vi "PIV_Pixel.vi"(8 "error in (no error)":errorcluster, 11 "PIV params":T2={"t"=path "/Users/crogers/Desktop/PIV/ezgif-split/frame_0_delay-0.14s.jpg", "t + dt"=path "/Users/crogers/Desktop/PIV/ezgif-split/frame_1_delay-0.14s.jpg", "PIV params"={"window size"=32, "search size"=38, "overlap"=17}}) -> (0 "error out":errorcluster={"status"=TRUE, "code"=1671, "source"="Python Node in PIV_Pixel.vi->LabVIEW_GUI.vi<APPEND>\n\nModule Path: /Users/crogers/Desktop/PIV/LabVIEW/subs/code.py\nFunction Name: piv\nPython returned the following error: <class 'OSError'>\nImageIO does not generally support reading folders. Limited support may be available via specific plugins. Specify the plugin explicitly using the `plugin` kwarg, e.g. `plugin='DICOM'`\n\n\n Call Stack information:\n['Traceback (most recent call last):\n', '  File \"/Users/crogers/Desktop/PIV/LabVIEW/subs/code.py\", line 8, in piv\n    frame_a = tools.imread(path_t)\n', '  File \"/Users/crogers/Library/Python/3.10/lib/python/site-packages/openpiv/tools.py\", line 337, in imread\n    im = _imread(filename)\n', '  File \"/Users/crogers/Library/Python/3.10/lib/python/site-packages/imageio/v3.py\", line 53, in imread\n    with imopen(uri, \"r\", **plugin_kwargs) as img_file:\n', '  File \"/Users/crogers/Library/Python/3.10/lib/python/site-packages/imageio/core/imopen.py\", line 223, in imopen\n    raise err_type(err_msg)\n', \"OSError: ImageIO does not generally support reading folders. Limited support may be available via specific plugins. Specify the plugin explicitly using the `plugin` kwarg, e.g. `plugin='DICOM'`\n\"]"}, 3 "pixels":T1={"x"=[[249.30535937373418, 248.42902364889454, 249.76279948299583, 247.41594341275038, 249.1115257279782, 247.78798944960093, 250.12043012406355, 247.87808352883224, 248.34885972253088, 249.7914207911112, 247.77762730848636, 249.1512614353793, 249.75511132386535, 250.2039453992136, 251.0671966033442, 249.57524164043096], [250.3340434377881, 250.00147110119926, 248.9863350898821, 248.5777445935735, 248.8999381795624, 248.0999411317878, 250.1052613689504, 248.91784014699442, 248.86156436587453, 250.04009873380096, 249.0256554262938, 248.65809383974363, 249.6866801516841, 250.34192499126266, 248.82795554993143, 249.0061437567773], [249.8379771192706, 249.42545268743535, 249.99132868734347, 248.92736756105637, 248.81643484942745, 249.3310863564142, 250.15105027103033, 249.12989134088602, 249.04454959724643, 247.59519201729674, 249.25833529503674, 247.47331898457645, 248.1888431064803, 250.79040549336878, 249.4526081113374, 249.6336800524876], [248.6980668234578, 248.54570865688697, 246.7725657136647, 249.35812326520707, 248.89034255886847, 246.4523690408173, 250.0452232403072, 249.550444871314, 249.9765476901514, 248.7568049322972, 248.6401612231491, 249.79883085797923, 249.40130797289405, 246.5629890714208, 247.80685370459122, 248.80462667572783], [250.01488921592187, 250.09153234704317, 248.9121711813194, 249.0997960432928, 248.23464430329008, 248.5390445092607, 250.14199554538584, 249.79526944527598, 249.15547166133257, 248.42913742312317, 248.66649765678002, 249.98783358463044, 249.3122662178276, 247.46275715637935, 247.09281127164536, 249.14196469060883], [248.4814726325146, 250.32578418378327, 252.73547131633674, 249.2578741433366, 248.12604140003066, 249.92341822045444, 250.0776499368854, 248.399064003398, 246.77201099675497, 248.27129179389703, 250.55497705596306, 249.65928326586936, 249.59825543346153, 247.44042616526, 248.20411140311407, 248.28014466979678], [248.00737255317583, 250.54707211705906, 249.21162645077857, 248.25886125408834, 248.0387539726566, 248.9153012638658, 250.18519850567776, 247.22467702968024, 249.76466629672095, 249.2556306748364, 250.02396374442702, 249.65051950062963, 250.4965660861888, 248.0925292927269, 248.91946592643953, 248.2637943515181], [246.1821494594906, 249.33082934098553, 248.94094393264493, 249.04158620653422, 249.26011732344762, 249.6661630920858, 248.34537482290315, 249.32958002145983, 248.44306056595542, 249.60284556401166, 249.11509294896507, 249.91933165248471, 248.13237489941073, 250.05627478689743, 248.8303136103349, 249.21198396258842], [247.40937679664955, 249.75749896985545, 248.32387807731334, 248.95535998273797, 250.07904312089906, 248.94164695256754, 247.77049810385864, 247.87385923341975, 248.15868824776928, 249.5424691779508, 248.67114136119247, 248.60481452263753, 247.09329148360536, 250.04657782089552, 247.76622030389302, 249.74825372082137], [248.40649315075004, 249.50680197039077, 249.01580784201263, 248.08513546511418, 250.23552350579513, 248.0561485178251, 249.0645116452157, 248.95113258123106, 251.75665115657733, 249.3997539918615, 248.66201521458854, 248.85160979570387, 248.38535817779288, 248.46760230981192, 247.46861084204957, 249.0122244330493], [249.14754561374613, 251.02569476688643, 249.8361169122564, 247.93392565584398, 249.95930525996766, 248.6162386371012, 249.08361536717862, 249.87630209464092, 249.48931646095573, 249.14607663576936, 248.62804527022283, 249.4249745322186, 248.7380918318621, 249.3604159325276, 248.72143788477564, 249.21304894216297], [248.35312686069207, 249.58820056157424, 248.3560103286516, 249.56629318575628, 249.59362672842414, 249.60331244219543, 249.10441364055487, 248.7328086777035, 248.89866953363116, 247.97866927062663, 249.3307073073744, 250.2239182398913, 249.16142037868028, 249.0563871396553, 249.4949006882887, 249.51436619145983]], "y"=[[0.8977283953687021, 0.6341863158832339, 0.9906547908510532, 3.106737289418504, 1.1821140984592304, 0.3751409283520246, 1.3818005864610683, -0.600121285455657, 0.6357268023560181, 0.845736566623323, -0.3731915769522587, -2.199033492516911, -0.21423581669690606, -0.3347594797784126, 1.1698087519270928, 1.566926374462696], [0.8965659508572088, 1.9437460996389433, 0.6224521757415502, -0.7217534453584307, 1.2037735939395944, 3.040914323466559, -0.3832771542393587, 0.15343686298088244, 0.997187747340611, 1.0527446150261355, 1.509697354230255, -2.1701091702073683, -2.2892314742890107, -0.6124409762401584, 1.25779577345142, 2.435950520643182], [-0.020908984575918055, 0.808132754103319, 1.5727649641668506, -0.45296926287363704, -1.208464478259863, -0.506959993186129, -0.5947669843271441, -0.975848708630167, -0.6421905816051066, -0.3987990096717908, -1.4070992684436234, -2.261505865838487, 0.06639054799464361, -1.1695814137185678, -0.3675269379222357, -0.2648923594257724], [0.3109771407276085, 0.5159494570786904, -1.4163299456319223, 0.07102651210981747, -1.2851252719297435, 0.10599760454645946, 0.7367107969054487, -0.16784210153293344, 0.27284316723275026, 0.4596314702594029, -0.4132105382968376, 2.593889260250748, 0.45294607371371143, -1.933834795200795, -1.0096684879789208, -0.15903235101450974], [0.23855007598676536, -1.9955308986860487, -1.3984666925978217, 0.48058552946130817, -0.015174367898751484, -0.7671366273104496, -0.8535820787912485, -0.7955505153384834, -1.017646873453515, -0.16739074452090108, 0.3648306981711258, 0.9307679362089871, 1.562958664327141, -0.04485662689486247, -0.23357418783209738, -0.6035663171106265], [0.013829448925584131, -1.9358349688371135, -1.4695962162198484, 0.5947964198860234, 0.2776392219589141, -0.22785775633131777, -0.15131917925703675, -0.4153649199674092, 0.4466333336464956, 0.25066493260030853, 0.35528947786236387, 1.3103000240386464, -0.2140304542018967, 0.12133392372160046, -0.49735044708949516, -0.2563433389042302], [2.0066903381980694, 2.794937422495103, 1.3981438682431957, 1.32543349324159, 0.022886535372457217, -0.9432851645218676, 0.0465564365104143, -0.9851058035259541, 0.8804035526296161, 1.2072293754869179, 0.42874909844545783, 1.7652653432293164, 0.47987536243230267, 0.26211844447008303, 0.6477767135804058, 1.191164256120203], [2.1410994418467055, 1.1177174463222528, 1.6983097882253162, 0.7617018915272666, 1.8895481438185868, -2.3308329687965923, 0.44458370084541343, 3.4411635098964055, 0.4202762082936573, -0.7767577642360024, -0.35753351457277205, -0.3741674249379656, 0.22728149074637827, -0.08923809505407831, 0.6029678418080664, 1.8102033968000697], [0.40552532193807167, 0.38050416917148056, 2.9728620478863377, 0.5848556588837539, 0.034000271349654554, -1.0697151619861955, -0.789201625615199, 0.3424590331110977, -0.014991496301952623, 0.1816448684692773, 0.16450838718995442, -0.8527519183298082, 0.5973103946411484, -0.21929086910912332, -0.2522634668837398, -0.5496729535634515], [-1.0784341723001134, 0.6385179489532433, 0.2624355393884059, 0.7800818345774729, -0.20223131443852793, -0.8799262477261038, 1.0814261425313276, 0.01896169162503014, -1.4323416215907159, -1.1447899618840296, 1.2953715679074662, 1.8011306347966993, -3.59547558301756, -1.51425732727688, -0.3005536713368784, -0.8495876802721014], [-0.48529100956749005, 3.7535484211289827, 0.4716731565341803, -0.16691798810644087, -1.3274681438865343, 1.4127784125875564, 2.503009927378308, 0.6744977470081182, 0.6289537982436144, 0.5592686551672443, -0.4793140551587527, 0.8966787006954746, 2.8181705852389882, 0.8982376832276984, 0.8024882650817133, 0.36402627005394095], [0.3348076271773692, 0.5833426717044787, 0.6325826470115814, -1.2167231134881717, 0.2408720624673677, -0.5408144273093995, 0.061549655902659595, 0.1198560631205936, 0.4155138438417083, -0.07385728581841278, 1.0016705373303125, -0.8491469124310314, -1.0571250384478148, 0.27765360370057834, 1.3863896930917718, 1.2780985374410747]], "u"=[[3.654057076523203, 3.906689254019018, 4.3499249727354785, 2.9769797253005232, 4.1985261262312195, 4.53911201630744, 3.6142265703335354, 4.545410360329742, 4.275176542616173, 3.9800504580894107, 3.945780644550432, 4.142828981573519, 3.997707165543276, 2.9923959435801497, 3.4106969202636495, 4.999245369266826], [4.721876610704807, 2.7791735544418565, 4.04797726724709, 3.1329268783475097, 4.706557050441488, 4.762468241690385, 3.039882623852986, 5.037812189846022, 3.357303836725008, 3.4488968279603935, 3.924508990313546, 4.201571037936669, 4.017913649448239, 4.3435322093850495, 4.387257019168252, 3.9180399717234993], [4.511693109203351, 3.6612724986035223, 4.269814446623989, 4.218697651581058, 4.807320057264706, 4.009377669328912, 4.405847778900064, 4.123688871016016, 3.784958247444461, 3.721978603867669, 4.353352122442394, 3.440608423789492, 4.8110182227292855, 3.909255097098531, 2.9020670167480147, 3.9050361810819143], [3.40465714069752, 3.9326981284321607, 4.0120727049173555, 3.7856505254893382, 3.7262750849724515, 2.9831152945719106, 3.7097179258624338, 4.35106035811602, 3.688332772188065, 3.747091966193779, 4.11025427675998, 3.9656181661692327, 2.9327313456835538, 4.150277635628887, 3.3765339532142065, 4.153106429159354], [3.387574609047479, 2.7699051515052755, 4.107458409125639, 4.471004094839486, 3.630386589969853, 3.7522818291832034, 4.592562274282968, 4.942019544439905, 3.6758264536017187, 5.090556637656444, 4.392992010857408, 3.7361463084414557, 2.644273868496813, 4.235012879773729, 4.017292315069722, 4.615785073786853], [4.845808184377554, 4.439541657576462, 2.897607886694547, 3.4661358674422065, 4.114576567616225, 4.2981580154498165, 4.45289017699371, 3.1067911933459214, 3.9731156019297735, 4.967565161826359, 4.274648262718975, 3.340537457109602, 4.007790619783492, 3.0484698597456186, 3.0902877440316217, 3.46977172973948], [4.105784905034725, 4.367232594403088, 3.4482894359240186, 3.519447403701663, 4.1592118776098825, 4.452636112938493, 4.402274236537246, 3.8791091835025098, 4.280101204874112, 4.097948666253696, 3.7883707470561188, 4.824890734154082, 4.952756144044697, 4.431182097404486, 4.243449943530994, 4.838679874357956], [3.400017358160556, 4.131421512821141, 4.1341151479233815, 3.868056363739919, 4.114722937313372, 3.182209432540521, 4.614370434260993, 4.411780339295759, 3.7355216305789054, 4.594274939159283, 4.491351839228378, 4.3193175610411325, 3.9283857185683773, 4.793911290126535, 4.649497598758955, 4.3396642398318335], [3.516007589124258, 4.196871268766618, 3.1728676439509176, 3.420084255337708, 4.592612630487026, 3.4822313601511596, 4.212353707965761, 5.4044957155037405, 4.095326795337716, 4.74614522754851, 5.01002718991552, 4.34430597630962, 4.3788685927631015, 4.9484451474366296, 3.6714296162586293, 3.410028692944248], [4.114243758496789, 3.342175456154506, 4.0764258974027605, 3.7136810067221804, 4.477618301281832, 4.208710770028269, 4.001606540014744, 3.657763910976016, 3.8103669626271897, 4.458090941819041, 3.891518974609637, 4.030571187954858, 2.728773248181442, 4.326154268416609, 4.733378911855885, 4.609860862498076], [3.7273513628033554, 2.4461192162266197, 3.9403444180392935, 4.236797064872377, 3.5225832678408047, 3.9117408717259883, 3.788069871625027, 4.554181400594344, 3.475295946618708, 3.288247776778453, 4.779964981541216, 3.6684037998946164, 3.1969710305814667, 3.7169385489979185, 3.872757705734433, 3.64012465662325], [3.4516528893089995, 4.387557930694406, 3.994367234165161, 4.086502040222127, 3.302726609880943, 4.115138490819219, 4.143240057429105, 4.669707669133866, 3.7284189048703174, 4.039756580842941, 2.557244072683501, 3.6402231851260347, 4.066441820254696, 4.519502569432314, 4.11575653582123, 4.385562395092346]], "v"=[[21.0, 42.0, 63.0, 84.0, 105.0, 126.0, 147.0, 168.0, 189.0, 210.0, 231.0, 252.0, 273.0, 294.0, 315.0, 336.0], [21.0, 42.0, 63.0, 84.0, 105.0, 126.0, 147.0, 168.0, 189.0, 210.0, 231.0, 252.0, 273.0, 294.0, 315.0, 336.0], [21.0, 42.0, 63.0, 84.0, 105.0, 126.0, 147.0, 168.0, 189.0, 210.0, 231.0, 252.0, 273.0, 294.0, 315.0, 336.0], [21.0, 42.0, 63.0, 84.0, 105.0, 126.0, 147.0, 168.0, 189.0, 210.0, 231.0, 252.0, 273.0, 294.0, 315.0, 336.0], [21.0, 42.0, 63.0, 84.0, 105.0, 126.0, 147.0, 168.0, 189.0, 210.0, 231.0, 252.0, 273.0, 294.0, 315.0, 336.0], [21.0, 42.0, 63.0, 84.0, 105.0, 126.0, 147.0, 168.0, 189.0, 210.0, 231.0, 252.0, 273.0, 294.0, 315.0, 336.0], [21.0, 42.0, 63.0, 84.0, 105.0, 126.0, 147.0, 168.0, 189.0, 210.0, 231.0, 252.0, 273.0, 294.0, 315.0, 336.0], [21.0, 42.0, 63.0, 84.0, 105.0, 126.0, 147.0, 168.0, 189.0, 210.0, 231.0, 252.0, 273.0, 294.0, 315.0, 336.0], [21.0, 42.0, 63.0, 84.0, 105.0, 126.0, 147.0, 168.0, 189.0, 210.0, 231.0, 252.0, 273.0, 294.0, 315.0, 336.0], [21.0, 42.0, 63.0, 84.0, 105.0, 126.0, 147.0, 168.0, 189.0, 210.0, 231.0, 252.0, 273.0, 294.0, 315.0, 336.0], [21.0, 42.0, 63.0, 84.0, 105.0, 126.0, 147.0, 168.0, 189.0, 210.0, 231.0, 252.0, 273.0, 294.0, 315.0, 336.0], [21.0, 42.0, 63.0, 84.0, 105.0, 126.0, 147.0, 168.0, 189.0, 210.0, 231.0, 252.0, 273.0, 294.0, 315.0, 336.0]], "Sig2noise"=[[24.0, 24.0, 24.0, 24.0, 24.0, 24.0, 24.0, 24.0, 24.0, 24.0, 24.0, 24.0, 24.0, 24.0, 24.0, 24.0], [45.0, 45.0, 45.0, 45.0, 45.0, 45.0, 45.0, 45.0, 45.0, 45.0, 45.0, 45.0, 45.0, 45.0, 45.0, 45.0], [66.0, 66.0, 66.0, 66.0, 66.0, 66.0, 66.0, 66.0, 66.0, 66.0, 66.0, 66.0, 66.0, 66.0, 66.0, 66.0], [87.0, 87.0, 87.0, 87.0, 87.0, 87.0, 87.0, 87.0, 87.0, 87.0, 87.0, 87.0, 87.0, 87.0, 87.0, 87.0], [108.0, 108.0, 108.0, 108.0, 108.0, 108.0, 108.0, 108.0, 108.0, 108.0, 108.0, 108.0, 108.0, 108.0, 108.0, 108.0], [129.0, 129.0, 129.0, 129.0, 129.0, 129.0, 129.0, 129.0, 129.0, 129.0, 129.0, 129.0, 129.0, 129.0, 129.0, 129.0], [150.0, 150.0, 150.0, 150.0, 150.0, 150.0, 150.0, 150.0, 150.0, 150.0, 150.0, 150.0, 150.0, 150.0, 150.0, 150.0], [171.0, 171.0, 171.0, 171.0, 171.0, 171.0, 171.0, 171.0, 171.0, 171.0, 171.0, 171.0, 171.0, 171.0, 171.0, 171.0], [192.0, 192.0, 192.0, 192.0, 192.0, 192.0, 192.0, 192.0, 192.0, 192.0, 192.0, 192.0, 192.0, 192.0, 192.0, 192.0], [213.0, 213.0, 213.0, 213.0, 213.0, 213.0, 213.0, 213.0, 213.0, 213.0, 213.0, 213.0, 213.0, 213.0, 213.0, 213.0], [234.0, 234.0, 234.0, 234.0, 234.0, 234.0, 234.0, 234.0, 234.0, 234.0, 234.0, 234.0, 234.0, 234.0, 234.0, 234.0], [255.0, 255.0, 255.0, 255.0, 255.0, 255.0, 255.0, 255.0, 255.0, 255.0, 255.0, 255.0, 255.0, 255.0, 255.0, 255.0]]})   [LabVIEW 2025]
uses:
  PIV_params.ctl
  PIV_velocities.ctl
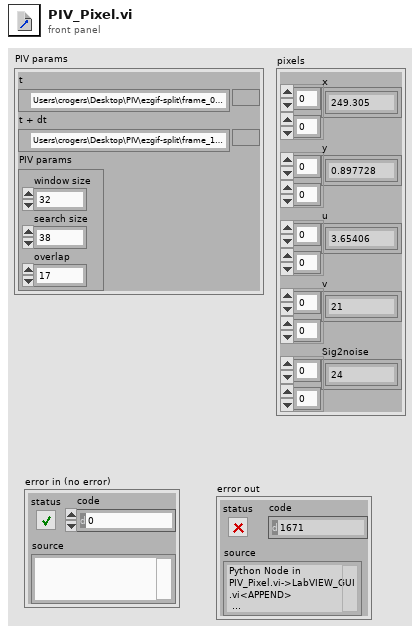
[diagram p1: front panel]
types:
  T1 = typedef "PIV_velocities.ctl" = cluster{"x":dbl[][], "y":dbl[][], "u":dbl[][], "v":dbl[][], "Sig2noise":dbl[][]}
  T2 = typedef "PIV_params.ctl" = cluster{"t":path, "t + dt":path, "PIV params":cluster{"window size":i16, "search size":i16, "overlap":i16}}
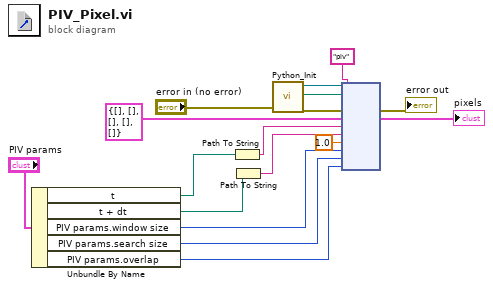
[diagram p0: block diagram]
diagram:
  n1 = Unbundle By Name("PIV params") -> ("t"=w5:path, "t + dt"=w4:path, "PIV params.window size"=w9:i16, "PIV params.search size"=w8:i16, "PIV params.overlap"=w7:i16)
  n2 = Path To String(path=w5) -> (string=w11:string)
  n3 = Path To String(path=w4) -> (string=w10:string)
  n4 = call "Python_Init.vi"("error in (no error)"="error in (no error)") -> ("Refnum out"=w16:refnum<k35>, "code"=w13:path, "error out"=w17:errorcluster)  [unwired: 3 in]
  n5 = node(w16, w13, "piv" ("function name"), w17, T1 {"x"=[], "y"=[], "u"=[], "v"=[], "Sig2noise"=[]} ("velocities"), w11, w10, 1.0 ("input parameter"), w9, w8, w7) -> (→"error out":errorcluster, →"pixels":T1)  [unwired: 6 in, 3 out]
